vi "LIA Fgen Dual Channel.vi"() -> ()   [LabVIEW 2017]
doc: "This example shows how to use the Arbitrary Waveform mode to generate on two channels."
uses:
  <instrlib>/niFgen/niFgen.llb/niFgen Output Mode.ctl
  <instrlib>/niFgen/niFgen.llb/niFgen Waveform Type.ctl
panel:
  in  "Vp 1":dbl=2.0 format="%_8g"
  in  "Frequency":dbl=100000.0 format="%_6p"
  in  "Vp 0":dbl=2.0 format="%_8g"
  in  "Stop":bool
  in  "FGEN Resource Name":refnum<k15>="Dev2"
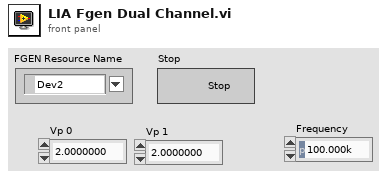
[diagram p1: front panel]
types:
  T1 = typedef "niFgen Waveform Type.ctl" = i32
  T2 = typedef "niFgen Output Mode.ctl" = u32
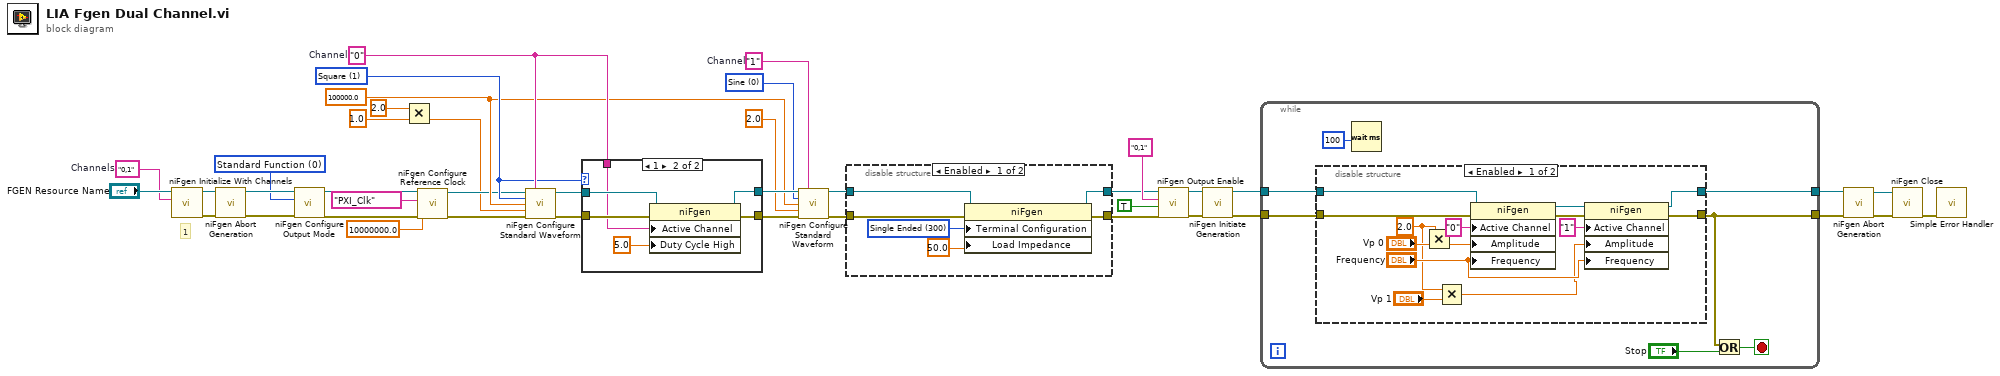
[diagram p0: block diagram]
diagram:
  w19 = "1"  # Channel
  w21 = T1 0 items=["Sine", "Square", "Triangle", "Ramp Up", "Ramp Down", "DC", "Noise", "User"] ("Waveform")
  w8 = 100000.0 ("Frequency")
  w9 = T1 1 items=["Sine", "Square", "Triangle", "Ramp Up", "Ramp Down", "DC", "Noise", "User"] ("Waveform")
  w26 = "0"  # Channel
  w32 = T2 0 items=["Standard Function", "Frequency List", "Arbitrary Waveform", "Arbitrary Sequence", "Script"] ("Output Mode")
  w37 = "0,1"  # Channels
  # "1"
  n1 = call <instrlib>:"niFgen Initialize With Channels.vi"("Channel Name"=w37, "Resource Name"="FGEN Resource Name") -> ("error out"=w36:errorcluster, "Instrument Handle Out"=w35:refnum<k15>)  [unwired: 8 in]
  n2 = call <instrlib>:"niFgen Abort Generation.vi"("error in (no error)"=w36, "Instrument Handle"=w35) -> ("error out"=w34:errorcluster, "Instrument Handle Out"=w33:refnum<k15>)  [unwired: 8 in]
  n3 = call <instrlib>:"niFgen Configure Output Mode.vi"("error in (no error)"=w34, "Output Mode (default: 0=Standard Function)"=w32, "Instrument Handle"=w33) -> ("error out"=w28:errorcluster, "Instrument Handle Out"=w6:refnum<k15>)  [unwired: 6 in]
  n4 = Multiply(x=2.0 ("Amplitude"), y=1.0 ("Amplitude")) -> (x*y=w2:dbl)
  n5 = call <instrlib>:"niFgen Configure Reference Clock.vi"("error in (no error)"=w28, "Reference Clock Frequency"=10000000.0, "Source"="PXI_Clk", "Instrument Handle"=w6) -> ("error out"=w7:errorcluster, "Instrument Handle Out"=w5:refnum<k15>)  [unwired: 6 in]
  n6 = call <instrlib>:"niFgen Configure Standard Waveform.vi"("Instrument Handle"=w5, "Channel Name"=w26, "Waveform"=w9, "Frequency"=w8, "Amplitude"=w2, "error in (no error)"=w7) -> ("Instrument Handle Out"=w30:refnum<k15>, "error out"=w29:errorcluster)  [unwired: 8 in]
  n7 = case shown="1" w9 {
    tunnel: w30 -> [w43 w49]
    tunnel: w29 -> [w42 w48]
    tunnel: w26 -> [_ w47]
    tunnel: [w43 w45] -> w22
    tunnel: [w42 w44] -> w18
    frame Default {
    }
    frame 1 {
      n8 = property class="niFgen"(reference=w49, error in=w48, "Active Channel"=w47, "Duty Cycle High"=5.0 ("Standard Function:Duty Cycle High")) -> (reference out=w45:refnum<k15>, error out=w44:errorcluster)
    }
  }
  n9 = call <instrlib>:"niFgen Configure Standard Waveform.vi"("Instrument Handle"=w22, "Channel Name"=w19, "Waveform"=w21, "Frequency"=w8, "Amplitude"=2.0, "error in (no error)"=w18) -> ("Instrument Handle Out"=w11:refnum<k15>, "error out"=w17:errorcluster)  [unwired: 8 in]
  n10 = disable-structure shown="Enabled" {
    disable-tunnel: w17 -> [w55 w56]
    disable-tunnel: [w54 w56] -> w12
    disable-tunnel: w11 -> [w53 w57]
    disable-tunnel: [w52 w57] -> w10
    frame Enabled {
      w51 = 300 items=["Single Ended"=300, "Differential"=301] ("Output:Terminal Configuration")
      n11 = property class="niFgen"(reference=w53, error in=w55, "Terminal Configuration"=w51, "Load Impedance"=50.0 ("Output:Load Impedance")) -> (reference out=w52:refnum<k15>, error out=w54:errorcluster)
    }
    frame Disabled {
    }
  }
  n12 = call <instrlib>:"niFgen Output Enable.vi"("error in (no error)"=w12, "Output Enable (default: True)"=TRUE ("output enable"), "Channel Name"="0,1", "Instrument Handle"=w10) -> ("error out"=w23:errorcluster, "Instrument Handle Out"=w24:refnum<k15>)  [unwired: 6 in]
  n13 = call <instrlib>:"niFgen Initiate Generation.vi"("error in (no error)"=w23, "Instrument Handle"=w24) -> ("error out"=w15:errorcluster, "Instrument Handle Out"=w13:refnum<k15>)  [unwired: 8 in]
  n14 = while {
    tunnel: [w60] -> w16
    tunnel: w15 -> [w61]
    tunnel: [w58] -> w14
    tunnel: w13 -> [w59]
    stop <- w62 stop-if-true
    n15 = disable-structure shown="Enabled" {
      disable-tunnel: w61 -> [w78 w79]
      disable-tunnel: [w73 w79] -> w60
      disable-tunnel: w59 -> [w76 w80]
      disable-tunnel: [w71 w80] -> w58
      frame Enabled {
        w66 = 2.0 ("x")
        n16 = Multiply(x=w66, y="Vp 0") -> (x*y=w68:dbl)
        n17 = Multiply(x=w66, y="Vp 1") -> (x*y=w65:dbl)
        n18 = property class="niFgen"(reference=w76, error in=w78, "Active Channel"="0", "Amplitude"=w68, "Frequency"="Frequency") -> (reference out=w72:refnum<k15>, error out=w77:errorcluster)
        n19 = property class="niFgen"(reference=w72, error in=w77, "Active Channel"="1", "Amplitude"=w65, "Frequency"="Frequency") -> (reference out=w71:refnum<k15>, error out=w73:errorcluster)
      }
      frame Disabled {
      }
    }
    n20 = Wait (ms)(milliseconds to wait=u32 100 ("millisecond multiple")) -> ()  [unwired: 1 out]
    n21 = Or(x=w60, y="Stop") -> (x .or. y?=w62:bool)
  }
  n22 = call <instrlib>:"niFgen Abort Generation.vi"("error in (no error)"=w16, "Instrument Handle"=w14) -> ("error out"=w41:errorcluster, "Instrument Handle Out"=w40:refnum<k15>)  [unwired: 8 in]
  n23 = call <instrlib>:"niFgen Close.vi"("error in (no error)"=w41, "Instrument Handle"=w40) -> ("error out"=w39:errorcluster)  [unwired: 9 in]
  n24 = call <vilib>:"Simple Error Handler.vi"("error in (no error)"=w39) -> ()  [unwired: 4 in, 5 out]
